vi "Connect OPC UA.vi"(6 "Sequence Context":refnum<k7>, 7 "OPC Ref Name":string, 8 "error in":errorcluster, 9 "Trial Number":i32=3, 10 "timeout(s)":T2=5, 11 "URL":string="opc.tcp://DESKTOP-T6QR0HI:4991/LunarTester") -> (0 "error out":errorcluster={"status"=TRUE, "code"=97, "source"="Unknown System Error in TestStand - Initialize Termination Monitor.vi->Login Progress.vi"})   [LabVIEW 2019, in "OPC UA.lvlib" / "OPC UA.lvclass"]
uses:
  OPC UA.lvclass
  <vilib>/OPCUA/controls/Time Out.ctl
  <vilib>/OPCUA/NI OPC UA Client.lvlib
panel:
  out "Connect":bool
  out "Note":string="Connecting to OPC Server"
  out "Waiting Lights":T1
  out "Trial":i32
  out "stop":bool
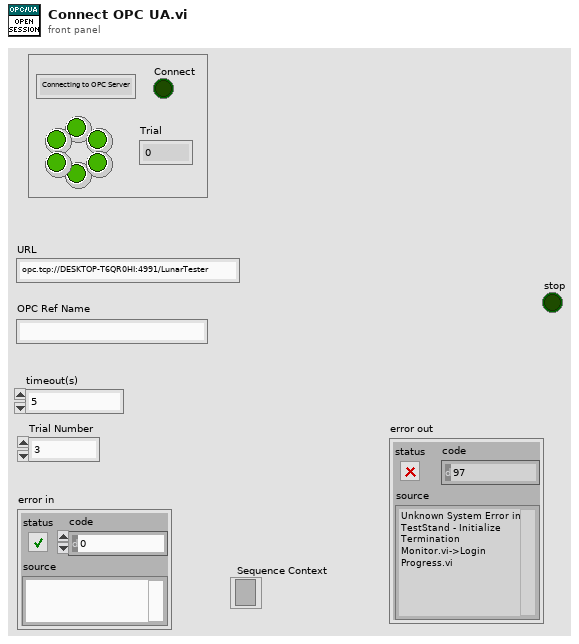
[diagram p1: front panel]
types:
  T1 = cluster{"wait 1":bool, "wait 2":bool, "wait 3":bool, "wait 4":bool, "wait 5":bool, "wait 6":bool}
  T2 = typedef "Time Out.ctl" = u32
  T3 = typedef "TestStand - Status Monitor.ctl" = cluster{"Sequence Context":refnum<k7>, "Execution":refnum<k7>, "Termination Monitor":refnum<k7>}
  T4 = cluster{"[0]":bool, "[1]":bool, "[2]":bool, "[3]":bool, "[4]":bool, "[5]":bool}
  T5 = typedef "OPC UA Client Refnum.ctl" = refnum<k21>
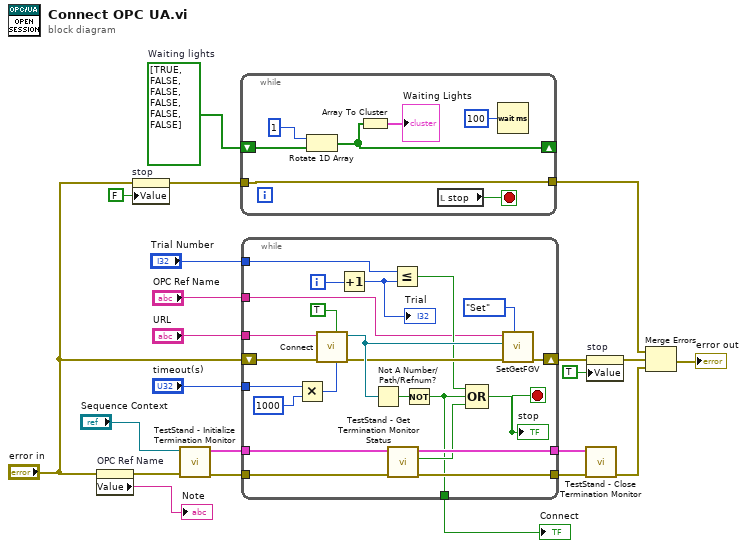
[diagram p0: block diagram]
diagram:
  w13 = bool[] [TRUE, FALSE, FALSE, FALSE, FALSE, FALSE]  # Waiting lights
  n1 = property on="OPC Ref Name" class="Str"(error in="error in") -> (error out=w6:errorcluster, "Value"=→"Note":string)  [unwired: 1 in, 1 out]
  n2 = property on="stop" class="Bool (strict)"(error in="error in", "Value"=FALSE ("stop")) -> (error out=w12:errorcluster)  [unwired: 1 in, 1 out]
  n3 = call <vilib>:"TestStand - Initialize Termination Monitor.vi"("error in (no error)"=w6, "Sequence Context In"="Sequence Context") -> ("error out"=w17:errorcluster, "Status Monitor Out"=w18:T3)  [unwired: 8 in]
  n4 = while {
    tunnel: w12 -> [w27]
    tunnel: [w27] -> w11
    shift-right: [w24] -> _
    shift-left: w13 -> [w25]
    stop <- w28 stop-if-true
    n5 = Rotate 1D Array(1:w25, 2:1 ("n")) -> (0:w24:bool[])
    n6 = Array To Cluster(array=w24) -> (cluster=→"Waiting Lights":T4)
    n7 = local read "stop"() -> (w28:bool)
    n8 = Wait (ms)(milliseconds to wait=u32 100) -> ()  [unwired: 1 out]
  }
  n9 = while {
    tunnel: "URL" -> [w50]
    tunnel: w17 -> [w46]
    tunnel: w18 -> [w47]
    tunnel: [w45] -> w19
    tunnel: [w44] -> w20
    tunnel: "timeout(s)" -> [w42]
    shift-right: [w43] -> w4
    shift-left: "error in" -> [w51]
    tunnel: "OPC Ref Name" -> [w33]
    tunnel: "Trial Number" -> [w31]
    tunnel: [w30] -> w1
    i -> [w39]
    stop <- w32 stop-if-true
    n10 = Multiply(x=w42, y=T2 1000) -> (x*y=w41:T2)
    n11 = call <vilib>:"Connect.vi"("timeout (5000 ms)"=w41, "trust any server (F)"=TRUE, "error in (no error)"=w51, "server endpoint URL"=w50) -> ("error out"=w37:errorcluster, "OPC UA client refnum out"=w48:T5)  [unwired: 5 in, 1 out]
    n12 = Increment(x=w39) -> (x+1=w38:i32)
    "Trial" <- w38
    n13 = Not A Number/Path/Refnum?(number/path/refnum=w48) -> (NaN/Path/Refnum?=w36:bool)
    n14 = call <vilib>:"TestStand - Get Termination Monitor Status.vi"("error in (no error)"=w46, "Status Monitor In"=w47) -> ("error out"=w44:errorcluster, "Terminating or Aborting"=w34:bool, "Status Monitor Out"=w45:T3)  [unwired: 7 in]
    n15 = Less Or Equal?(x=w31, y=w38) -> (x <= y?=w35:bool)
    n16 = Not(x=w36) -> (.not. x?=w30:bool)
    n17 = Compound Arithmetic op=OR(w35, w30, w34) -> (w32:bool)
    "stop" <- w32
    n18 = call "SetGetFGV.vi"("Method (Get)"=enum16{"Get", "Set"}."Set", "error in"=w37, "Data In"=w48, "Name"=w33) -> ("error out"=w43:errorcluster)  [unwired: 6 in, 1 out]
  }
  "Connect" <- w1
  n19 = call <vilib>:"TestStand - Close Termination Monitor.vi"("error in (no error)"=w20, "Status Monitor In"=w19) -> ("error out"=w21:errorcluster)  [unwired: 9 in]
  n20 = property on="stop" class="Bool (strict)"(error in=w4, "Value"=TRUE ("stop")) -> (error out=w3:errorcluster)  [unwired: 1 in, 1 out]
  n21 = Merge Errors(w11, w3, w21) -> (→"error out":errorcluster)
